vi "Write StateCompleted.vi"(8 "error in (no error)":errorcluster, 10 "StateCompleted":bool, 11 "State in":refnum<class "State.lvclass">) -> (0 "error out":errorcluster, 3 "State out":refnum<class "State.lvclass">)   [LabVIEW 2013, in "State.lvclass"]
uses:
  State.lvclass
  State.lvclass/State.ctl
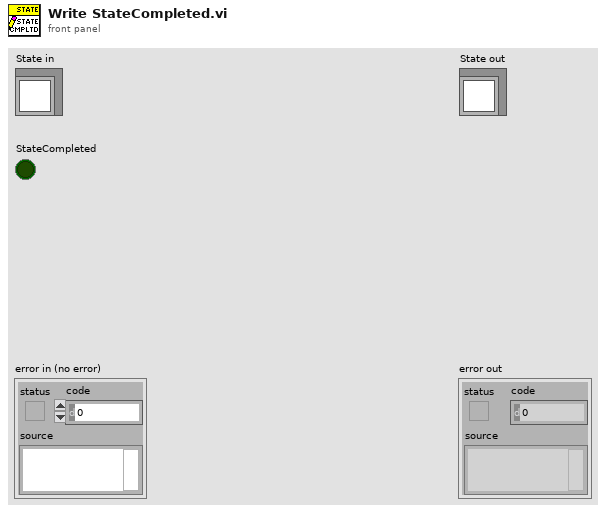
[diagram p1: front panel]
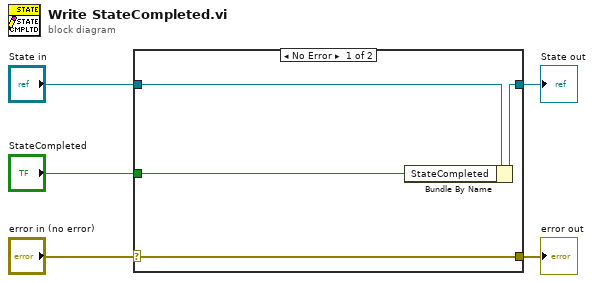
[diagram p0: block diagram]
diagram:
  n1 = case shown="No Error" "error in (no error)" {
    selector: "error in (no error)" -> [w9 w10]
    tunnel: [w9 w10] -> w4
    tunnel: [w7 w11] -> w2
    tunnel: "State in" -> [w8 w11]
    tunnel: "StateCompleted" -> [w6 _]
    frame No Error {
      n2 = Bundle By Name(cluster=w8, "StateCompleted"=w6) -> (w7:refnum<class "State.lvclass">)
    }
    frame Error {
    }
  }
  "error out" <- w4
  "State out" <- w2
